vi "GetStringArray.vi"(11 "Sequence Context":refnum<k7>) -> (0 "error out":errorcluster)   [LabVIEW 2011]
doc: "Reads the string array data from the local variable using the TestStand API and displays it."
uses:
  <vilib>/addons/TestStand/_TSUtility.llb/TestStand - Get Property Value (String Array).vi
panel:
  out "Array":string[](array[string])
  in  "OK":bool
  # "String Array Data"
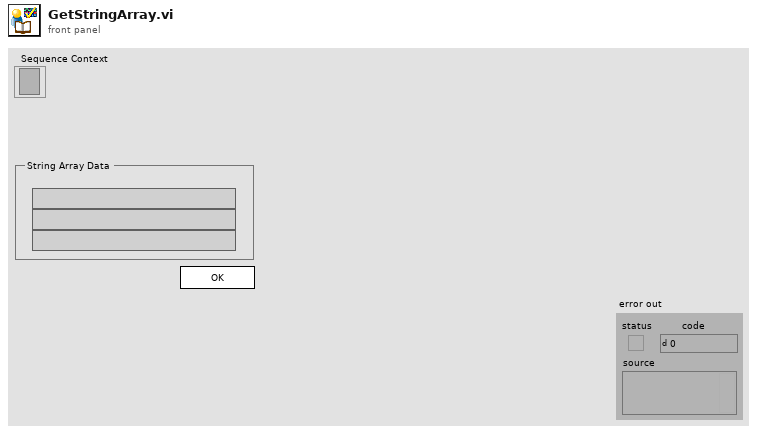
[diagram p1: front panel]
types:
  T1 = typedef "TestStand - Status Monitor.ctl" = cluster{"Sequence Context":refnum<k7>, "Execution":refnum<k7>, "Termination Monitor":refnum<k7>}
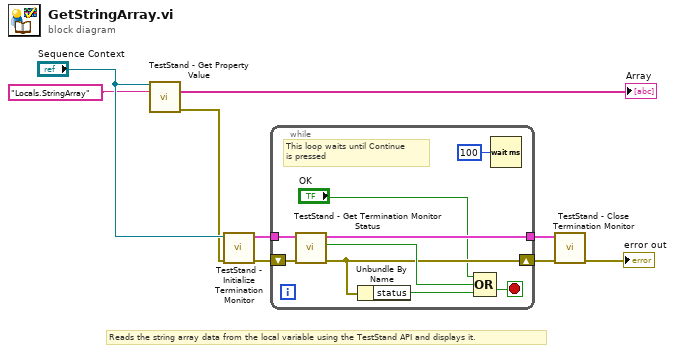
[diagram p0: block diagram]
diagram:
  # "Reads the string array data from the local variable using the TestStand API and displays it."
  n1 = call-poly <vilib>:"TestStand - Get Property Value.vi"("Sequence Context In"="Sequence Context", "Lookup String"="Locals.StringArray") -> ("Value"=→"Array":string[], "error out"=w6:errorcluster)  [unwired: 1 in, 11 out]
  n2 = call <vilib>:"TestStand - Initialize Termination Monitor.vi"("error in (no error)"=w6, "Sequence Context In"="Sequence Context") -> ("error out"=w3:errorcluster, "Status Monitor Out"=w5:T1)  [unwired: 8 out]
  n3 = while {
    shift-left: w3 -> [w16]
    shift-right: [w13] -> w2
    tunnel: [w17] -> w4
    tunnel: w5 -> [w18]
    stop <- w15 stop-if-true
    # "This loop waits until Continue \nis pressed"
    n4 = call <vilib>:"TestStand - Get Termination Monitor Status.vi"("error in (no error)"=w16, "Status Monitor In"=w18) -> ("error out"=w13:errorcluster, "Terminating or Aborting"=w14:bool, "Status Monitor Out"=w17:T1)  [unwired: 7 out]
    n5 = Unbundle By Name(w13) -> ("status"=w12:bool)
    n6 = Compound Arithmetic op=OR("OK", w14, w12) -> (w15:bool)
    n7 = Wait (ms)(milliseconds to wait=u32 100) -> ()  [unwired: 1 out]
  }
  n8 = call <vilib>:"TestStand - Close Termination Monitor.vi"("error in (no error)"=w2, "Status Monitor In"=w4) -> ("error out"=→"error out":errorcluster)  [unwired: 9 out]
